vi "Init Data.vi"(8 "error in (no error)":errorcluster, 10 "Data Object":refnum<class "Factory Plugin Framework.lvclass">, 11 "Generic DUT Setup in":refnum<class "Generic DUT Setup.lvclass">) -> (0 "error out":errorcluster, 3 "Generic DUT Setup out":refnum<class "Generic DUT Setup.lvclass">)   [LabVIEW 2018, in "Generic DUT Setup.lvlib" / "Generic DUT Setup.lvclass"]
uses:
  Generic DUT Setup.lvclass
  Plugins/FPF.lvlibp/Factory Plugin Framework.lvclass
  Plugins/Measurement Interface.lvlibp/Measurement Interface.lvclass
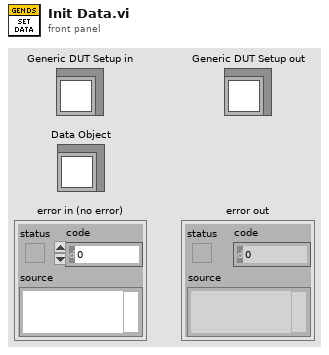
[diagram p1: front panel]
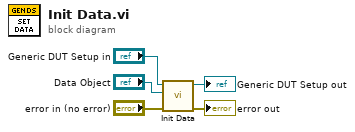
[diagram p0: block diagram]
diagram:
  n1 = call-parent "Init Data.vi"("error in (no error)"="error in (no error)", "Data Object"="Data Object", "Measurement Interface in"="Generic DUT Setup in") -> ("error out"=→"error out":errorcluster, "Measurement Interface out"=→"Generic DUT Setup out":refnum<class "Generic DUT Setup.lvclass">)  [unwired: 7 in]
